vi "FlowSensorCheckForTimeout.vi"(11 "FlowSensorSampleSensorLoopData in":T1={"State"=enum."WaitForTrigger", "StateAfterRead"=enum."ClearRxFIFO", "Timestamp"=0, "Timeout"=0, "U32"=0, "CRC"=0, "Exception"=0, "Sample"={"Timestamp"=0, "TxBytes"=0, "RxBytes"=0, "TxFrames"=0, "RxFrames"=0, "SignalStrength"=0, "FlowRate"=0, "NetTotalizer"=0, "PositiveTotalizer"=0, "NegativeTotalizer"=0, "Temperature1"=0, "Temperature2"=0}, "ErrorSample"={"Timestamp"=0, "TxBytes"=0, "RxBytes"=0, "TxFrames"=0, "RxFrames"=0, "ErrorCode"=enum."None"}}) -> (3 "FlowSensorSampleSensorLoopData out":T1={"State"=enum."WaitForTrigger", "StateAfterRead"=enum."ClearRxFIFO", "Timestamp"=0, "Timeout"=0, "U32"=0, "CRC"=0, "Exception"=0, "Sample"={"Timestamp"=0, "TxBytes"=0, "RxBytes"=0, "TxFrames"=0, "RxFrames"=0, "SignalStrength"=0, "FlowRate"=0, "NetTotalizer"=0, "PositiveTotalizer"=0, "NegativeTotalizer"=0, "Temperature1"=0, "Temperature2"=0}, "ErrorSample"={"Timestamp"=0, "TxBytes"=0, "RxBytes"=0, "TxFrames"=0, "RxFrames"=0, "ErrorCode"=enum."None"}})   [LabVIEW 2018]
uses:
  FlowSensorSampleSensorLoopData.ctl
  FlowSensorSampleSensorLoopStates.ctl
  FlowSensorSample.ctl
  FlowSensorErrorSample.ctl
  FlowSensorErrorCodes.ctl
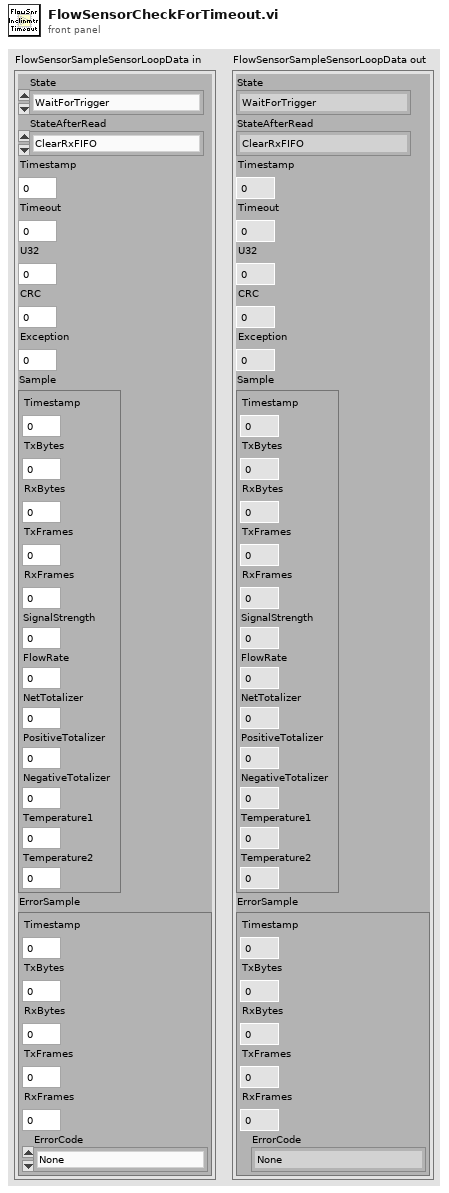
[diagram p1: front panel]
types:
  T1 = typedef "FlowSensorSampleSensorLoopData.ctl" = cluster{"State":T2, "StateAfterRead":T2, "Timestamp":u64, "Timeout":i32, "U32":u32, "CRC":u16, "Exception":u8, "Sample":T3, "ErrorSample":T4}
  T2 = typedef "FlowSensorSampleSensorLoopStates.ctl" = enum16{"WaitForTrigger", "ClearRxFIFO", "WaitForClearComplete", "WriteAddress", "WriteFunction", "WriteStartAddress1", "WriteStartAddress0", "WriteAddressCount1", "WriteAddressCount0", "WriteCRC1", "WriteCRC0", "ReadAddress", "ReadFunction", "ReadByteCount", "StartSignalStrength", "EndSignalStrength", "StartFlowRate", "EndFlowRate", "StartNetTotalizer", "EndNetTotalizer", "StartPositiveTotalizer", "EndPositiveTotalizer", "StartNegativeTotalizer", "EndNegativeTotalizer", "StartTemperature1", "EndTemperature1", "StartTemperature2", "EndTemperature2", "ReadDataByte1", "ReadDataByte0", "ReadDataByte3", "ReadDataByte2", "ReadCRCByte0", "ReadCRCByte1", "CalculateCRC", "ValidateCRC", "PrepareSample", "MoveSample", "ReadExceptionCode", "ReadExceptionCRCByte0", "ReadExceptionCRCByte1", "CalculateExceptionCRC", "ValidateExceptionCRC", "ParseExceptionCode", "ResponseAddressError", "ResponseFunctionCodeError", "ResponseByteCountError", "ResponseCRCError", "ResponseUnknownError", "ResponseTimeoutError", "SensorReportsIllegalFunction", "SensorReportsIllegalDataAddress", "PrepareErrorCode", "MoveErrorCode"}
  T3 = typedef "FlowSensorSample.ctl" = cluster{"Timestamp":u64, "TxBytes":u64, "RxBytes":u64, "TxFrames":u64, "RxFrames":u64, "SignalStrength":u32, "FlowRate":u32, "NetTotalizer":u32, "PositiveTotalizer":u32, "NegativeTotalizer":u32, "Temperature1":u32, "Temperature2":u32}
  T4 = typedef "FlowSensorErrorSample.ctl" = cluster{"Timestamp":u64, "TxBytes":u64, "RxBytes":u64, "TxFrames":u64, "RxFrames":u64, "ErrorCode":T5}
  T5 = typedef "FlowSensorErrorCodes.ctl" = enum8{"None", "ResponseAddressError", "ResponseFunctionCodeError", "ResponseByteCountError", "ResponseCRCError", "ResponseUnknownError", "ResponseTimeoutError", "SensorReportsIllegalFunction", "SensorReportsIllegalDataAddress"}
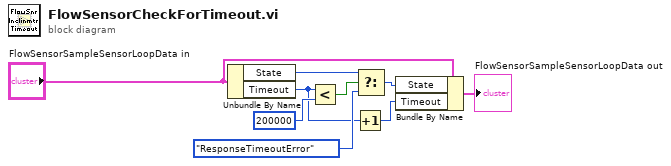
[diagram p0: block diagram]
diagram:
  n1 = Unbundle By Name("FlowSensorSampleSensorLoopData in") -> ("State"=w1:T2, "Timeout"=w4:i32)
  n2 = Less?(x=w4, y=200000) -> (x < y?=w7:bool)
  n3 = Increment(x=w4) -> (x+1=w9:i32)
  n4 = Select(t=w1, s=w7, f=FlowSensorSampleSensorLoopStates."ResponseTimeoutError" ("InclinometerState")) -> (s? t:f=w5:T2)
  n5 = Bundle By Name(cluster="FlowSensorSampleSensorLoopData in", "State"=w5, "Timeout"=w9) -> (→"FlowSensorSampleSensorLoopData out":T1)
